vi "test.vi"() -> ()   [LabVIEW 2019]
panel:
  out "Cluster 2":T1 {"Thermometer" scale=0.0..100.0}
  in  "Cluster":cluster{"Slide":dbl, "Boolean":bool} {"Slide" scale=0.0..100.0}
  in  "stop":bool
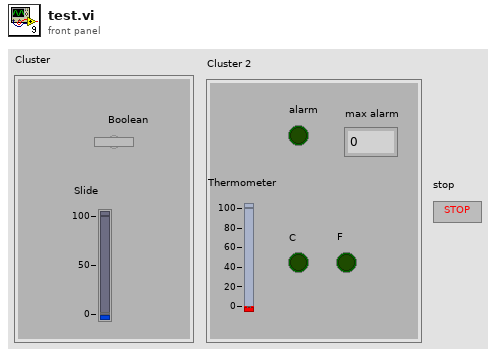
[diagram p1: front panel]
types:
  T1 = cluster{"Thermometer":dbl, "alarm":bool, "C":bool, "F":bool, "max alarm":dbl}
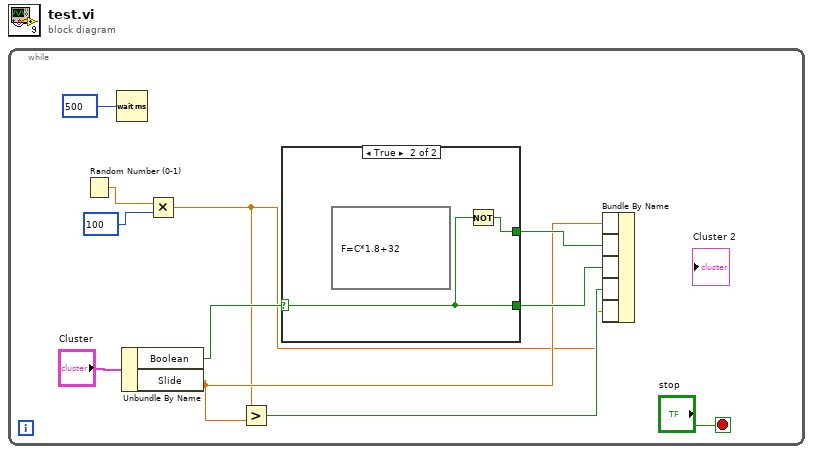
[diagram p0: block diagram]
diagram:
  n1 = while {
    stop <- "stop" stop-if-true
    n2 = Random Number (0-1)() -> (number: 0 to 1=w9:dbl)
    n3 = Wait (ms)(milliseconds to wait=500) -> ()  [unwired: 1 out]
    n4 = Unbundle By Name("Cluster") -> ("Boolean"=w6:bool, "Slide"=w2:dbl)
    n5 = Multiply(x=w9, y=100) -> (x*y=w1:dbl)
    n6 = Greater?(x=w1, y=w2) -> (0:w3:bool)
    n7 = case shown="True" w6 {
      selector: w6 -> [_ w12]
      tunnel: [_ w13] -> w5
      tunnel: [_ w12] -> w4
      frame False {
      }
      frame True {
        n8 = formula code="F=C*1.8+32"() -> ()
        n9 = Not(x=w12) -> (.not. x?=w13:bool)
      }
    }
    n10 = Bundle By Name(w2, w5, w4, w3, w1) -> ()  [unwired: 1 in, 1 out]
  }
